vi "Siglent SDS 1000 2000 Series Acquire Waveform With Preview.vi"() -> ()   [LabVIEW 2021]
doc: "This example shows how to use advanced waveform readout parameters. The Preview Waveform Data graph shows signal decimated based on First Point, Sparsing and Number Of Points parameters. The Full Waveform Data graph shows full data as they were acquired by the instrument.\nObserve the time it takes to download the preview data and the full data."
uses:
  <instrlib>/Siglent SDS 1000 2000 Series/Siglent SDS 1000 2000 Series.lvlib
panel:
  in  "Number Of Points (0: all points)":i32
  in  "First Point (0: first point)":i32
  out "Full Download Time  (ms)":u32
  out "Full Waveform Data":waveform(dbl)(graph)
  in  "Sparsing (1000)":i32=1000
  out "Preview Download Time  (ms)":u32
  in  "Vertical Coupling (0: A1M)":u16(ring) items=["A1M", "A50", "D1M", "D50", "Ground"]
  in  "Probe Attenuation (1X)":dbl=1.0
  in  "Vertical Range (1 V)":dbl=1.0
  in  "Timebase (0.0005 s)":dbl=0.0005
  out "Preview Waveform Data":waveform(dbl)(graph)
  in  "Source (1: Channel 1)":u16(ring)=1 items=["Channel 1"=1, "Channel 2"=2, "Channel 3"=3, "Channel 4"=4]
  in  "VISA resource name":refnum<visa-resource-name>
  # "(c) 2015 SIGLENT TECHNOLOGIES CO., LTD.   ALL RIGHTS RESERVED."
  # "Note:\nThis VI will time out without acquiring any data if the input signal on the selected channel does not cross 0 V trigger level with positive slope."
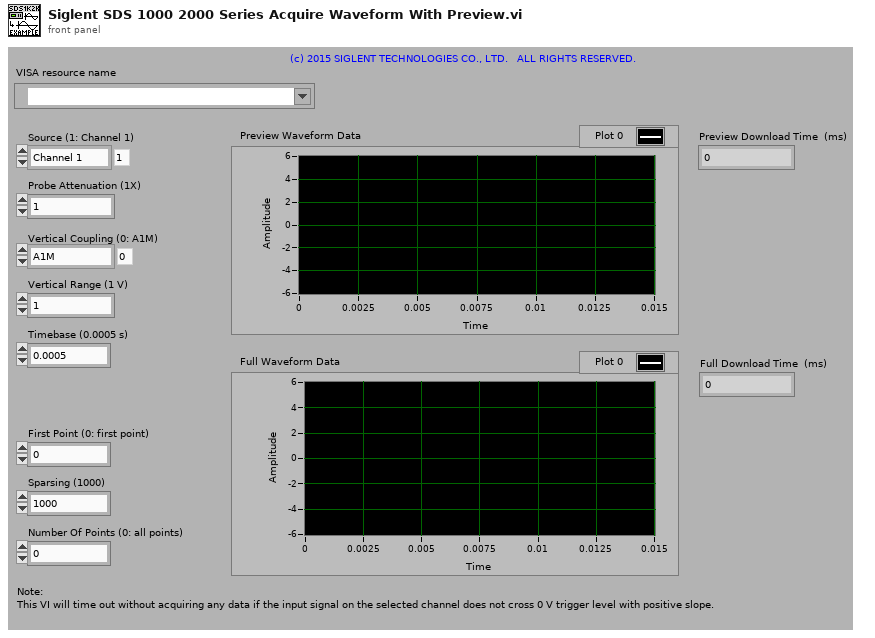
[diagram p1: front panel]
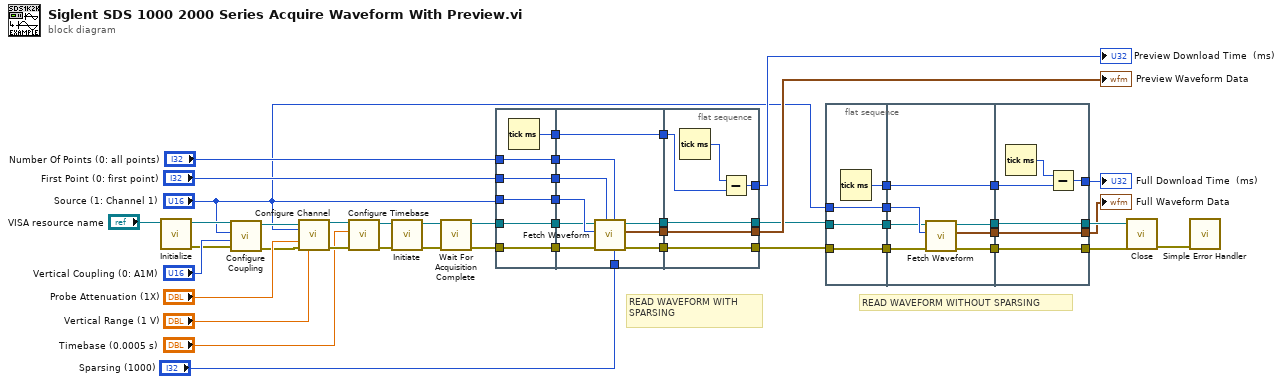
[diagram p0: block diagram]
diagram:
  # "READ WAVEFORM WITHOUT SPARSING"
  # "READ WAVEFORM WITH SPARSING"
  n1 = call <instrlib>:"Initialize.vi"("VISA resource name"="VISA resource name") -> ("error out"=w2:errorcluster, "VISA resource name out"=w5:refnum<visa-resource-name>)  [unwired: 9 in]
  n2 = call <instrlib>:"Configure Coupling.vi"("error in (no error)"=w2, "Vertical Coupling (0: A1M)"="Vertical Coupling (0: A1M)", "Channel (1: Channel 1)"="Source (1: Channel 1)", "VISA resource name"=w5) -> ("error out"=w3:errorcluster, "VISA resource name out"=w4:refnum<visa-resource-name>)  [unwired: 6 in]
  n3 = call <instrlib>:"Configure Channel.vi"("VISA resource name"=w4, "Channel (1: Channel 1)"="Source (1: Channel 1)", "Probe Attenuation (1X)"="Probe Attenuation (1X)", "error in (no error)"=w3, "Vertical Range (1.0 V)"="Vertical Range (1 V)") -> ("VISA resource name out"=w46:refnum<visa-resource-name>, "error out"=w47:errorcluster)  [unwired: 9 in]
  n4 = call <instrlib>:"Configure Timebase.vi"("error in (no error)"=w47, "Timebase (0.0005 s)"="Timebase (0.0005 s)", "VISA resource name"=w46) -> ("error out"=w12:errorcluster, "VISA resource name out"=w11:refnum<visa-resource-name>)  [unwired: 7 in]
  n5 = call <instrlib>:"Initiate.vi"("error in (no error)"=w12, "VISA resource name"=w11) -> ("error out"=w10:errorcluster, "VISA resource name out"=w9:refnum<visa-resource-name>)  [unwired: 8 in]
  n6 = call <instrlib>:"Wait For Acquisition Complete.vi"("error in (no error)"=w10, "VISA resource name"=w9) -> ("error out"=w7:errorcluster, "VISA resource name out"=w8:refnum<visa-resource-name>)  [unwired: 7 in, 1 out]
  n7 = flat-sequence {
    tunnel: "Source (1: Channel 1)" -> [w53]
    tunnel: [w53] -> w24
    tunnel: w8 -> [w52]
    tunnel: [w52] -> w23
    tunnel: w7 -> [w51]
    tunnel: [w51] -> w22
    tunnel: "First Point (0: first point)" -> [w50]
    tunnel: [w50] -> w21
    tunnel: [w54] -> w20
    tunnel: [w49] -> w14
    tunnel: "Number Of Points (0: all points)" -> [w49]
    tunnel: [w64] -> w19
    tunnel: w24 -> [w63]
    tunnel: w23 -> [w62]
    tunnel: w22 -> [w61]
    tunnel: [w60] -> w18
    tunnel: [w59] -> w17
    tunnel: w21 -> [w58]
    tunnel: w20 -> [w57]
    tunnel: [w57] -> w16
    tunnel: "Sparsing (1000)" -> [w56]
    tunnel: w14 -> [w55]
    tunnel: [w67] -> w43
    tunnel: w19 -> [w67]
    tunnel: [w69] -> w40
    tunnel: [w66] -> w39
    tunnel: w18 -> [w66]
    tunnel: [w65] -> w38
    tunnel: w17 -> [w65]
    tunnel: w16 -> [w70]
    frame #0 {
      n8 = Tick Count (ms)() -> (millisecond timer value=w54:u32)
    }
    frame #1 {
      n9 = call <instrlib>:"Fetch Waveform.vi"("Sparsing (0: Every point)"=w56, "Number of points (0: All points)"=w55, "First point (0: First point)"=w58, "error in (no error)"=w61, "Source (1: Channel 1)"=w63, "VISA resource name"=w62) -> ("error out"=w59:errorcluster, "Waveform Graph"=w64:waveform(dbl), "VISA resource name out"=w60:refnum<visa-resource-name>)  [unwired: 3 in]
    }
    frame #2 {
      n10 = Tick Count (ms)() -> (millisecond timer value=w68:u32)
      n11 = Subtract(x=w68, y=w70) -> (x-y=w69:u32)
    }
  }
  n12 = flat-sequence {
    tunnel: "Source (1: Channel 1)" -> [w73]
    tunnel: [w73] -> w32
    tunnel: w39 -> [w72]
    tunnel: [w72] -> w31
    tunnel: w38 -> [w71]
    tunnel: [w71] -> w30
    tunnel: [w74] -> w29
    tunnel: [w81] -> w28
    tunnel: w32 -> [w80]
    tunnel: w31 -> [w79]
    tunnel: w30 -> [w78]
    tunnel: [w77] -> w27
    tunnel: [w76] -> w26
    tunnel: w29 -> [w75]
    tunnel: [w75] -> w25
    tunnel: [w84] -> w35
    tunnel: w28 -> [w84]
    tunnel: [w86] -> w34
    tunnel: [w83] -> w37
    tunnel: w27 -> [w83]
    tunnel: [w82] -> w36
    tunnel: w26 -> [w82]
    tunnel: w25 -> [w87]
    frame #0 {
      n13 = Tick Count (ms)() -> (millisecond timer value=w74:u32)
    }
    frame #1 {
      n14 = call <instrlib>:"Fetch Waveform.vi"("error in (no error)"=w78, "Source (1: Channel 1)"=w80, "VISA resource name"=w79) -> ("error out"=w76:errorcluster, "Waveform Graph"=w81:waveform(dbl), "VISA resource name out"=w77:refnum<visa-resource-name>)  [unwired: 6 in]
    }
    frame #2 {
      n15 = Tick Count (ms)() -> (millisecond timer value=w85:u32)
      n16 = Subtract(x=w85, y=w87) -> (x-y=w86:u32)
    }
  }
  n17 = call <instrlib>:"Close.vi"("error in (no error)"=w36, "VISA resource name"=w37) -> ("error out"=w48:errorcluster)  [unwired: 9 in]
  n18 = call <vilib>:"Simple Error Handler.vi"("error in (no error)"=w48) -> ()  [unwired: 4 in, 5 out]
  "Preview Waveform Data" <- w43
  "Preview Download Time  (ms)" <- w40
  "Full Waveform Data" <- w35
  "Full Download Time  (ms)" <- w34
